vi "Start or stop continuous status updates.vi"(8 "error in (no error)":errorcluster, 10 "Continuous status updates":bool, 11 "PS Control Actor in":refnum<class "PS Control Actor.lvclass">) -> (0 "error out":errorcluster, 3 "PS Control Actor out":refnum<class "PS Control Actor.lvclass">)   [LabVIEW 2025, in "PS Control Actor.lvlib" / "PS Control Actor.lvclass"]
doc: "Author: Scott Hannahs <sth@magnet.fsu.edu>\n\nThis software is licensed for use under the “MIT License\"\nCopyright (c) 2025 Scott Hannahs, sth@sth@magnet.sthnet.net\n\nPermission is hereby granted, free of charge, to any person obtaining a copy of this software and associated documentation files (the \"Software\"), to deal in the Software without restriction, including without limitation the rights to use, copy, modify, merge, publish, distribute, sublicense, and/or sell copies of the Software, and to permit persons to whom the Software is furnished to do so, subject to the following conditions: The above copyright notice and this permission notice shall be included in all copies or substantial portions of the Software.\n\nTHE SOFTWARE IS PROVIDED \"AS IS\", WITHOUT WARRANTY OF ANY KIND, EXPRESS OR IMPLIED, INCLUDING BUT NOT LIMITED TO THE WARRANTIES OF MERCHANTABILITY, FITNESS FOR A PARTICULAR PURPOSE AND NONINFRINGEMENT. IN NO EVENT SHALL THE AUTHORS OR COPYRIGHT HOLDERS BE LIABLE FOR ANY CLAIM, DAMAGES OR OTHER LIABILITY, WHETHER IN AN ACTION OF CONTRACT, TORT OR OTHERWISE, ARISING FROM, OUT OF OR IN CONNECTION WITH THE SOFTWARE OR THE USE OR OTHER DEALINGS IN THE SOFTWARE."
uses:
  PS Control Actor.lvclass
  PS Control Actor.lvclass/PS Control Actor.ctl
  <vilib>/ActorFramework/Actor/Actor.lvclass/Actor.ctl
  <vilib>/ActorFramework/Message Enqueuer/Message Enqueuer.lvclass/Message Enqueuer.ctl
  <vilib>/ActorFramework/Message Enqueuer/Init from Existing Queue.vi
  <vilib>/ActorFramework/Message Enqueuer/Enqueue.vi
  PS Control Actor Messages/Get PS Status Msg/Get PS Status Msg.lvclass
  <vilib>/ActorFramework/Message Priority Queue/Priority Enqueue.vi
  <vilib>/ActorFramework/Message Enqueuer/Message Enqueuer.lvclass
  <vilib>/ActorFramework/Actor/Actor.lvclass
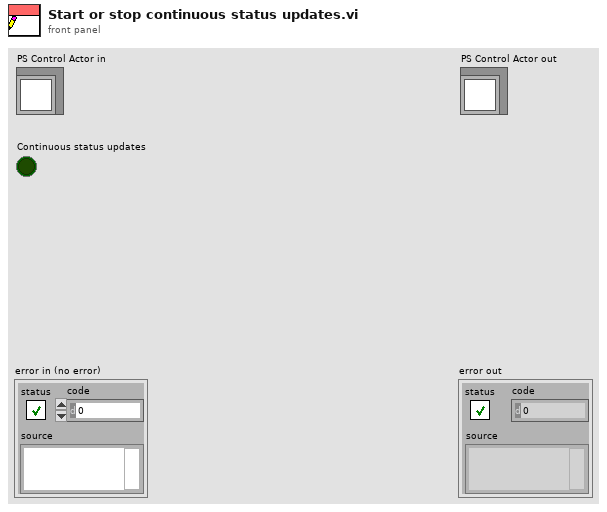
[diagram p1: front panel]
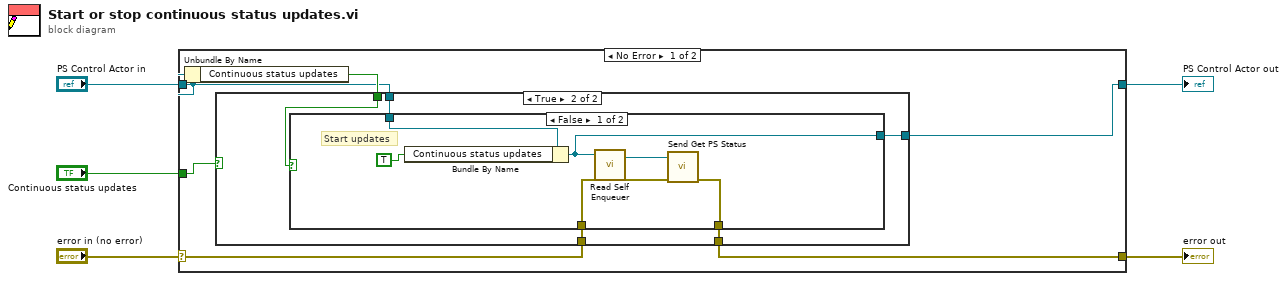
[diagram p0: block diagram]
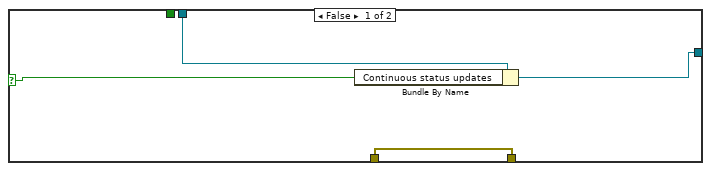
[diagram p2: hidden frame]
diagram:
  n1 = case shown="No Error" "error in (no error)" {
    selector: "error in (no error)" -> [w9 w29]
    tunnel: [w8 w29] -> w4
    tunnel: [w6 w30] -> w2
    tunnel: "PS Control Actor in" -> [w7 w30]
    tunnel: "Continuous status updates" -> [w11 _]
    frame No Error {
      n2 = Unbundle By Name(w7) -> ("Continuous status updates"=w10:bool)
      n3 = case shown="True" w11 {
        selector: w11 -> [w12 _]
        tunnel: w10 -> [_ w20]
        tunnel: w7 -> [w13 w19]
        tunnel: w9 -> [w15 w18]
        tunnel: [w15 w17] -> w8
        tunnel: [w14 w16] -> w6
        frame False {
          n4 = Bundle By Name(cluster=w13, "Continuous status updates"=w12) -> (w14:refnum<class "PS Control Actor.lvclass">)
        }
        frame True {
          n5 = case shown="False" w20 {
            tunnel: w19 -> [w23 w27]
            tunnel: w18 -> [w25 w28]
            tunnel: [w24 w28] -> w17
            tunnel: [w22 w27] -> w16
            frame False {
              # "Start updates"
              n6 = Bundle By Name(cluster=w23, "Continuous status updates"=TRUE) -> (w22:refnum<class "PS Control Actor.lvclass">)
              n7 = call <vilib>:"Read Self Enqueuer.vi"("Actor"=w22) -> ("Self Enqueuer"=w26:refnum<class "Message Enqueuer.lvclass">)  [unwired: 10 in]
              n8 = call "Send Get PS Status.vi"("error in (no error)"=w25, "Message Enqueuer"=w26) -> ("error out"=w24:errorcluster)  [unwired: 8 in, 1 out]
            }
            frame True {
              # "Already running. No change."
            }
          }
        }
      }
    }
    frame Error {
    }
  }
  "error out" <- w4
  "PS Control Actor out" <- w2
